vi "DEPRECATED DLL Initialize.vi"(8 "error in (no error)":errorcluster, 11 "Phasor Data Concentrator in":refnum<class "Phasor Data Concentrator.lvclass">) -> (0 "error out":errorcluster, 3 "Phasor Data Concentrator out":refnum<class "Phasor Data Concentrator.lvclass">)   [LabVIEW 2012]
doc: "Calls the DLL class to connect to the PDC."
uses:
  ABB C37.118 DLL/ABB C37.118 DLL.lvclass
  Phasor Data Concentrator.lvclass
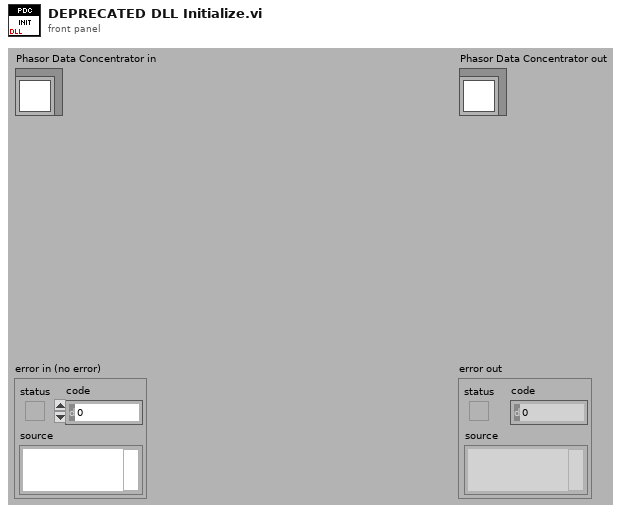
[diagram p1: front panel]
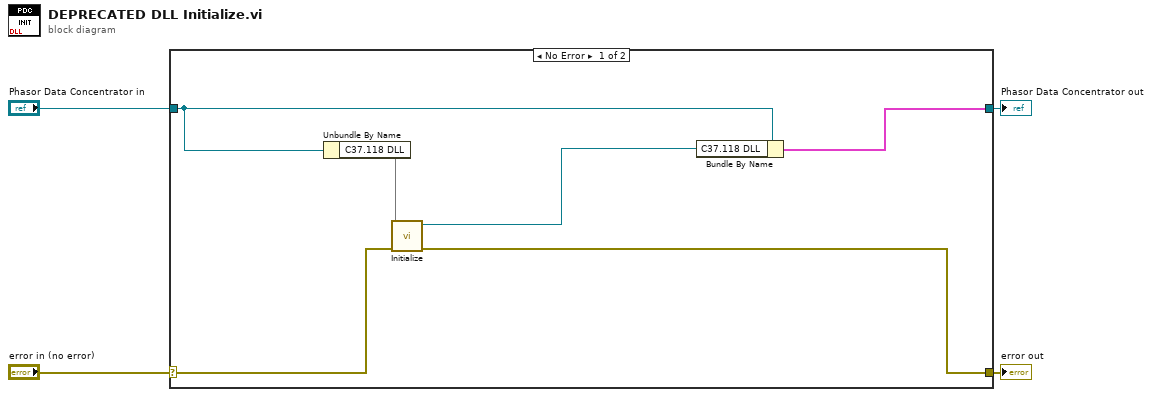
[diagram p0: block diagram]
diagram:
  n1 = case shown="No Error" "error in (no error)" {
    selector: "error in (no error)" -> [w8 w12]
    tunnel: [w5 w12] -> w3
    tunnel: [w6 w11] -> w1
    tunnel: "Phasor Data Concentrator in" -> [w9 w11]
    frame No Error {
      n2 = Unbundle By Name(w9) -> ("C37.118 DLL"=w10)
      n3 = call "Initialize.vi"("error in (no error)"=w8, "ABB C37.118 DLL in"=w10) -> ("error out"=w5:errorcluster, "ABB C37.118 DLL out"=w7:refnum<class "ABB C37.118 DLL.lvclass">)  [unwired: 8 in]
      n4 = Bundle By Name(cluster=w9, "C37.118 DLL"=w7) -> (w6:cluster{})
    }
    frame Error {
    }
  }
  "error out" <- w3
  "Phasor Data Concentrator out" <- w1
